vi "convertToKeyValuePair_1Dstring.vi"(8 "error in (no error)":errorcluster, 10 "value":string[](array[string]), 11 "name":string) -> (0 "error out":errorcluster, 3 "string converted":string)   [LabVIEW 2018]
doc: "Convert a 1-dimension string array into a key value pair as string."
uses:
  convertToKeyValuePair_string.vi
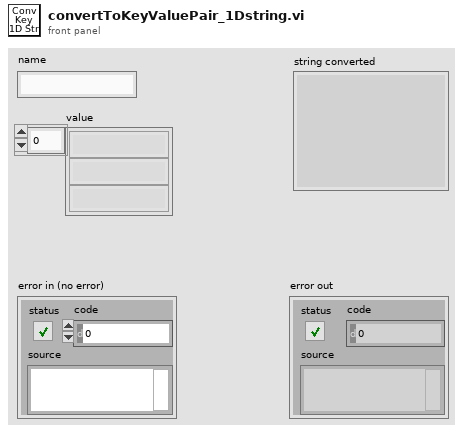
[diagram p1: front panel]
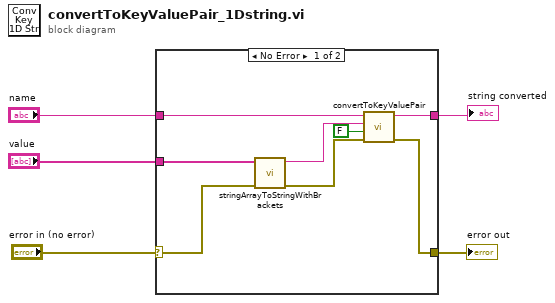
[diagram p0: block diagram]
diagram:
  n1 = case shown="No Error" "error in (no error)" {
    selector: "error in (no error)" -> [w7 w14]
    tunnel: "value" -> [w6 _]
    tunnel: "name" -> [w12 _]
    tunnel: [w11 w14] -> w2
    tunnel: [w13 _] -> w1
    frame No Error {
      n2 = call "stringArrayToStringWithBrackets.vi"("error in (no error)"=w7, "value"=w6) -> ("error out"=w9:errorcluster, "String"=w8:string)  [unwired: 8 in]
      n3 = call-poly "convertToKeyValuePair.vi"("error in (no error)"=w9, "double quotes (T)"=FALSE ("double quotes (F)"), "value"=w8, "name"=w12) -> ("error out"=w11:errorcluster, "string converted"=w13:string)  [unwired: 6 in]
    }
    frame Error {
    }
  }
  "error out" <- w2
  "string converted" <- w1
